vi "generateModels_v3.vi"() -> ()   [LabVIEW 2016]
panel:
  out "error IO":errorcluster
  in  "SCAN_NO":string="0000"
  in  "Process VSCAN":bool
  in  "stop":bool
  # "You can use any of these numbers for testing: \n2032, 2043"
  # ">>>"
  # ">> Script will automatically output the figure plot"
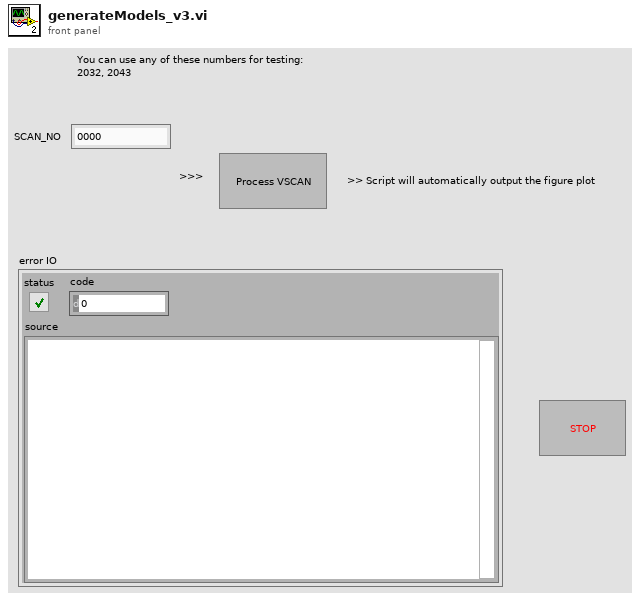
[diagram p1: front panel]
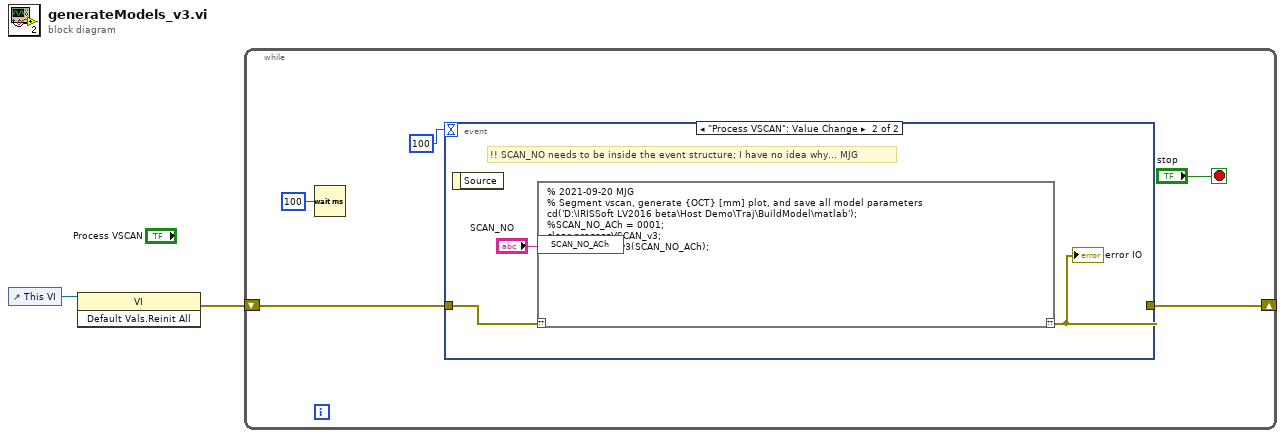
[diagram p0: block diagram]
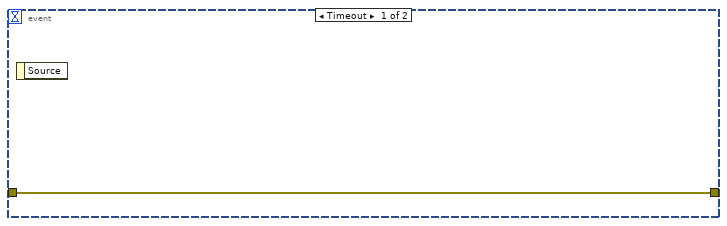
[diagram p2: hidden frame]
diagram:
  n1 = control-ref of="This VI"() -> (w1:refnum<vi>)
  n2 = invoke class="VI" method="Default Vals.Reinit All"(reference=w1) -> (error out=w2:errorcluster)  [unwired: 2 in, 2 out]
  n3 = while {
    shift-right: [w3] -> _
    shift-left: w2 -> [w5]
    stop <- "stop" stop-if-true
    n4 = Wait (ms)(milliseconds to wait=u32 100) -> ()  [unwired: 1 out]
    n5 = event shown="[1] \"Process VSCAN\": Value Change" {
      selector: _ -> [_ _]
      dyn-events: _ -> [_ _]
      timeout: 100 -> [_ _]
      tunnel: [w8 w10] -> w3
      tunnel: w5 -> [w8 w11]
      event Timeout {
        # "timeout"
        n6 = event-data() -> ()  [unwired: 1 in, 1 out]
      }
      event "Process VSCAN": Value Change {
        # "!! SCAN_NO needs to be inside the event structure; I have no idea why... MJG"
        # "run ML script to segment the vscan (ACh or PC)"
        n7 = event-data() -> ()  [unwired: 1 in, 1 out]
        n8 = script code="% 2021-09-20 MJG \n% Segment vscan, generate {OCT} [mm] plot, and save all model parameters\ncd('D:\\IRISSoft LV2016 beta\\Host Demo\\Traj\\BuildModel\\matlab');\n%SCAN_NO_ACh = 0001;\nclear processVSCAN_v3;\nprocessVSCAN_v3(SCAN_NO_ACh);" ("Script Node")("??"=w11, "SCAN_NO_ACh"="SCAN_NO") -> ("??"=w10:errorcluster)
        "error IO" <- w10
      }
    }
  }
